vi "FixFileName.vi"(9 "Filename":string) -> (4 "fixed filename":string, 5 "version":string)   [LabVIEW 2014, in "RasPiDownloader.lvlib"]
uses:
  RasPiDownloader.lvlib
  <vilib>/regexp/Match Regular Expression.xnode
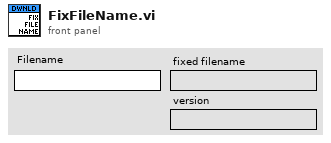
[diagram p1: front panel]
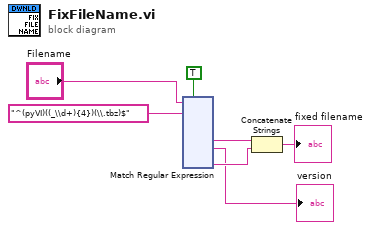
[diagram p0: block diagram]
diagram:
  n1 = xnode "Match Regular Expression"("input string"="Filename", "regular expression"="^(pyVI)((_\\d+){4})(\\.tbz)$", "ignore case? (F)"=TRUE) -> ("submatch 1"=w4:string, "submatch 2"=→"version":string, "submatch 4"=w2:string)  [unwired: 3 in, 6 out]
  n2 = Concatenate Strings(w4, w2) -> (→"fixed filename":string)
